vi "Simulate LVDT PointByPoint.vi"() -> ()   [LabVIEW 8.6]
uses:
  vi.lib/UeiDaq/UeiDaqConfigureTimingForSimpleIO.vi
  <libdir>/resource/objmgr/ueidaq.rc
  vi.lib/UeiDaq/UeiDaqWriteOneScaledScan.vi
panel:
  in  "Vrms":T1
  in  "Data Write Method":T2(ring)
  in  "Sensor Sensitivity":dbl
  in  "Simulated displacement":dbl(slide)
  in  "Excitation frequency":dbl
  in  "Excitation voltage":dbl
  in  "Wiring Scheme":enum16{"Four Wires", "Five wires"}(ring)
  in  "AO Resource":string
  in  "Refresh rate (ms)":u32
  in  "stop":bool
  # "Simulate LVDT"
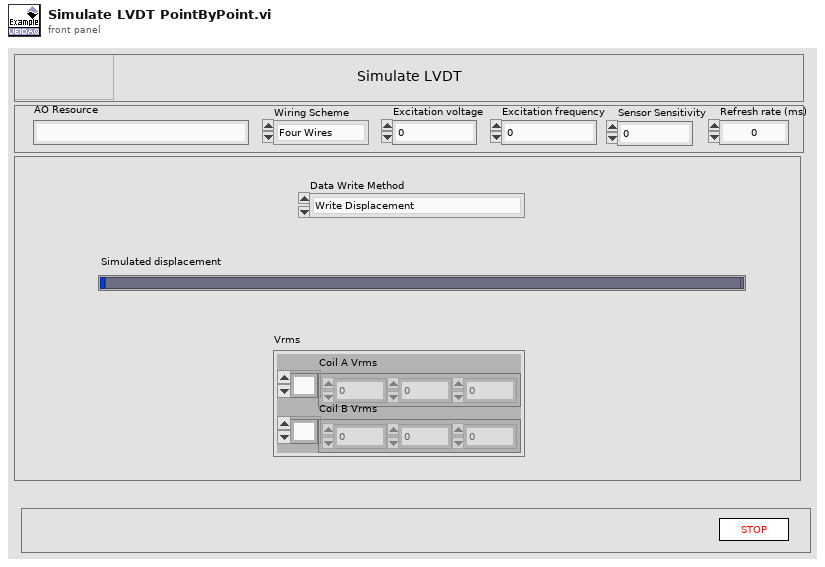
[diagram p1: front panel]
types:
  T1 = cluster{"Coil A Vrms":dbl[], "Coil B Vrms":dbl[]}
  T2 = enum16{"Write Displacement", "Write Coils Amplitudes", ""}
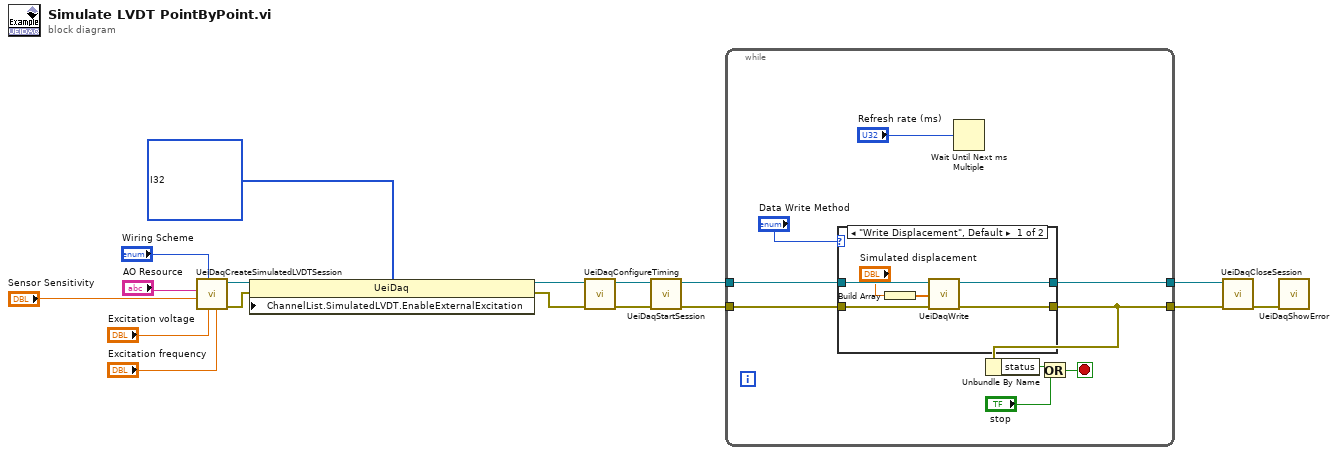
[diagram p0: block diagram]
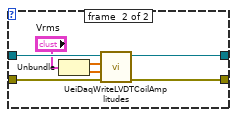
[diagram p2: hidden frame]
diagram:
  w6 = i32[] ? items=["Internal", "External"] ("Channel List:Simulated LVDT Output:Enable External Excitation")
  n1 = call "UeiDaqCreateSimulatedLVDTSession.vi"("Excitation frequency"="Excitation frequency", "Excitation voltage"="Excitation voltage", "Wiring Scheme"="Wiring Scheme", "Sensor Sensitivity"="Sensor Sensitivity", "Resource"="AO Resource") -> ("error out"=w8:errorcluster, "UeiDaq Refnum Out"=w10:refnum<k20>)  [unwired: 5 in]
  n2 = property class="UeiDaq"(reference=w10, error in=w8, "ChannelList.SimulatedLVDT.EnableExternalExcitation"=w6) -> (reference out=w9:refnum<k20>, error out=w7:errorcluster)
  n3 = call-poly "UeiDaqConfigureTiming.vi"("error in (no error)"=w7, "UeiDaq Refnum In"=w9) -> ("error out"=w2:errorcluster, "UeiDaq Refnum Out"=w4:refnum<k20>)  [unwired: 8 out]
  n4 = call "UeiDaqStartSession.vi"("error in (no error)"=w2, "UeiDaq Refnum In"=w4) -> ("error out"=w1:errorcluster, "UeiDaq Refnum Out"=w3:refnum<k20>)  [unwired: 8 in]
  n5 = while {
    tunnel: w3 -> [w20]
    tunnel: [w22] -> w16
    tunnel: w1 -> [w19]
    tunnel: [w21] -> w14
    stop <- w25 stop-if-true
    n6 = case shown="\"Write Displacement\", Default" "Data Write Method" {
      tunnel: [w29 w39] -> w22
      tunnel: [w31 w38] -> w21
      tunnel: w20 -> [w32 w37]
      tunnel: w19 -> [w30 w36]
      frame #0 {
        n7 = Build Array("Simulated displacement") -> (w27:dbl[])
        n8 = call-poly "UeiDaqWrite.vi"("error in (no error)"=w30, "Scaled Data"=w27, "UeiDaq Refnum In"=w32) -> ("error out"=w29:errorcluster, "UeiDaq Refnum Out"=w31:refnum<k20>)  [unwired: 7 in]
      }
      frame #1 {
        n9 = Unbundle("Vrms") -> ("Coil A Vrms"=w34:dbl[], "Coil B Vrms"=w33:dbl[])
        n10 = call "UeiDaqWriteLVDTCoilAmplitudes.vi"("UeiDaq Refnum In"=w37, "Primary coils Vrms"=w34, "Secondary coils Vrms"=w33, "error in (no error)"=w36) -> ("UeiDaq Refnum Out"=w38:refnum<k20>, "error out"=w39:errorcluster)  [unwired: 5 in]
      }
    }
    n11 = Wait Until Next ms Multiple(millisecond multiple="Refresh rate (ms)") -> ()  [unwired: 1 out]
    n12 = Unbundle By Name(w22) -> ("status"=w23:bool)
    n13 = Or(x=w23, y="stop") -> (x .or. y?=w25:bool)
  }
  n14 = call "UeiDaqCloseSession.vi"("error in (no error)"=w16, "UeiDaq Refnum In"=w14) -> ("error out"=w15:errorcluster)  [unwired: 1 in, 8 out]
  n15 = call "UeiDaqShowError.vi"("error in (no error)"=w15) -> ()  [unwired: 2 in, 9 out]
